vi "AlmostEqual_Abs_SGL.vi"(5 "X":sgl, 7 "Tolerance (Epsilon)":sgl=1.1920929e-07, 9 "Y":sgl) -> (8 "X = Y +/- Tolerance?":bool)   [LabVIEW 2020]
doc: "Determines if two double precision numbers are almost equal to eachother.\nTolerance parameter is the allowable absolute difference between the two numbers.\n\nNotes:\n- Use this function if you know the range of values to be compared. \n- Comparison to NaN will always return false.\n- Comparison to +/- Inf will always return false.\n\nSource: http://randomascii.wordpress.com/2012/02/25/comparing-floating-point-numbers-2012-edition/"
panel:
  # "Determines if two single precision numbers are almost equal to eachother.\nTolerance parameter is the allowable absolute difference between the two numbers.\n\nNotes:\n- Use this function if you know the range of values to be compared. \n- Comparison to NaN will always return false.\n- Comparison to +/- Inf will always return false."
  # "Source: http://randomascii.wordpress.com/2012/02/25/comparing-floating-point-numbers-2012-edition/"
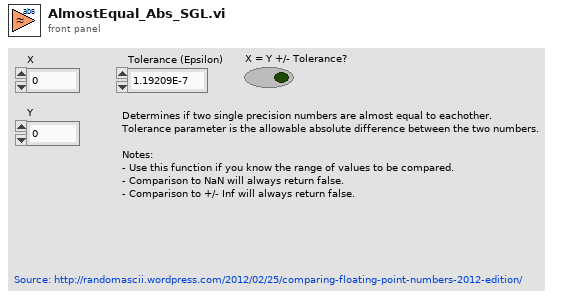
[diagram p1: front panel]
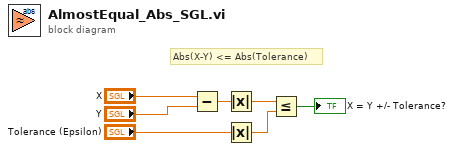
[diagram p0: block diagram]
diagram:
  # "Abs(X-Y) <= Abs(Tolerance)"
  n1 = Subtract(x="X", y="Y") -> (x-y=w5:sgl)
  n2 = Absolute Value(x=w5) -> (abs(x)=w3:sgl)
  n3 = Absolute Value(x="Tolerance (Epsilon)") -> (abs(x)=w1:sgl)
  n4 = Less Or Equal?(x=w3, y=w1) -> (x <= y?=→"X = Y +/- Tolerance?":bool)
